vi "FPGA_EncoderReadConfiguration.vi"(8 "error in (no error)":errorcluster, 11 "EncoderDevRef":T5) -> (0 "error out":errorcluster, 1 "BSource":T1={"DevStatus"={"status"=FALSE, "code"=0, "source"=""}, "AnalogTriggerMode?"=FALSE, "DigitalMode"={"DIO Channel"=enum."Disabled"}, "AnalogTriggerMode"={"AnalogTriggerIndex"=enum."Trig 0", "OutputType"=enum."InWindow"}}, 2 "ASource":T1={"DevStatus"={"status"=FALSE, "code"=0, "source"=""}, "AnalogTriggerMode?"=FALSE, "DigitalMode"={"DIO Channel"=enum."Disabled"}, "AnalogTriggerMode"={"AnalogTriggerIndex"=enum."Trig 0", "OutputType"=enum."InWindow"}}, 3 "EncoderDevRef":T5, 4 "Reverse?":bool, 5 "IndexSource":T1={"DevStatus"={"status"=FALSE, "code"=0, "source"=""}, "AnalogTriggerMode?"=FALSE, "DigitalMode"={"DIO Channel"=enum."Disabled"}, "AnalogTriggerMode"={"AnalogTriggerIndex"=enum."Trig 0", "OutputType"=enum."InWindow"}}, 6 "IndexActiveHigh":bool, 7 "Enable":bool)   [LabVIEW 2017]
uses:
  <vilib>/Rock Robotics/SystemInterfaces/Encoder/FPGA_EncoderDevRef.ctl
  <vilib>/Rock Robotics/SystemInterfaces/Encoder/FPGA_EncoderIdx.ctl
  <vilib>/Rock Robotics/SystemInterfaces/CounterEncoderSourceConvertion/FPGA_CounterEncoderSourceConvertionLVSourceType.ctl
  <vilib>/Rock Robotics/SystemInterfaces/DIO/FPGA_DIODigitalSourceChannel.ctl
  <vilib>/Rock Robotics/SystemInterfaces/AnalogTrigger/FPGA_AnalogTriggerIndex.ctl
  <vilib>/Rock Robotics/SystemInterfaces/AnalogTrigger/FPGA_AnalogTriggerOutType.ctl
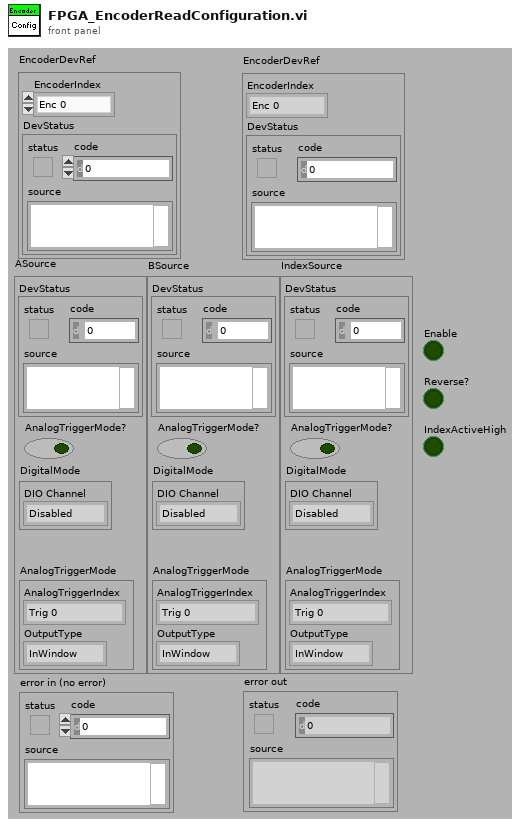
[diagram p1: front panel]
types:
  T1 = typedef "FPGA_CounterEncoderSourceConvertionLVSourceType.ctl" = cluster{"DevStatus":errorcluster, "AnalogTriggerMode?":bool, "DigitalMode":cluster{"DIO Channel":T2}, "AnalogTriggerMode":cluster{"AnalogTriggerIndex":T3, "OutputType":T4}}
  T2 = typedef "FPGA_DIODigitalSourceChannel.ctl" = enum8{"DIO 0", "DIO 1", "DIO 2", "DIO 3", "DIO 4", "DIO 5", "DIO 6", "DIO 7", "DIO 8", "DIO 9", "DIO MXP 0", "DIO MXP 1", "DIO MXP 2", "DIO MXP 3", "DIO MXP 4", "DIO MXP 5", "DIO MXP 6", "DIO MXP 7", "DIO MXP 8", "DIO MXP 9", "DIO MXP 10", "DIO MXP 11", "DIO MXP 12", "DIO MXP 13", "DIO MXP 14", "DIO MXP 15", "Disabled"}
  T3 = typedef "FPGA_AnalogTriggerIndex.ctl" = enum8{"Trig 0", "Trig 1", "Trig 2", "Trig 3", "Trig 4", "Trig 5", "Trig 6", "Trig 7", "Invalid"}
  T4 = typedef "FPGA_AnalogTriggerOutType.ctl" = enum16{"InWindow", "TriggerState", "Rising", "Falling"}
  T5 = typedef "FPGA_EncoderDevRef.ctl" = cluster{"EncoderIndex":T6, "DevStatus":errorcluster}
  T6 = typedef "FPGA_EncoderIdx.ctl" = enum8{"Enc 0", "Enc 1", "Enc 2", "Enc 3", "Enc 4", "Enc 5", "Enc 6", "Enc 7", "Invalid"}
  T7 = cluster{"ASource":cluster{"Channel":fxp<+,4,4>, "Module":fxp<+,1,1>, "AnalogTrigger":bool}, "BSource":cluster{"Channel":fxp<+,4,4>, "Module":fxp<+,1,1>, "AnalogTrigger":bool}, "IndexSource":cluster{"Channel":fxp<+,4,4>, "Module":fxp<+,1,1>, "AnalogTrigger":bool}, "IndexActiveHigh":bool, "Reverse":bool, "Enable":bool}
  T8 = cluster{"Channel":fxp<+,4,4>, "Module":fxp<+,1,1>, "AnalogTrigger":bool}
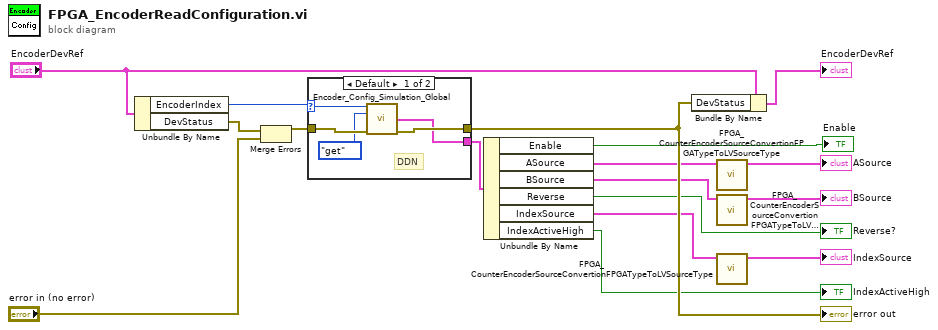
[diagram p0: block diagram]
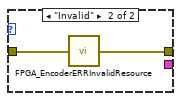
[diagram p2: hidden frame]
diagram:
  n1 = Unbundle By Name("EncoderDevRef") -> ("EncoderIndex"=w7:T6, "DevStatus"=w1:errorcluster)
  n2 = Merge Errors(w1, "error in (no error)") -> (w2:errorcluster)
  n3 = case shown="Default" w7 {
    selector: w7 -> [w22 _]
    tunnel: w2 -> [w21 w24]
    tunnel: [w20 w23] -> w14
    tunnel: [w19 _] -> w6
    frame Default {
      # "DDN"
      n4 = call <vilib>:"Encoder_Config_Simulation_Global.vi"("EncoderIndex"=w22, "menu"=enum16{"set", "get", "delete"}."get", "error in (no error)"=w21) -> ("Encoder Config get"=w19:T7, "error out"=w20:errorcluster)  [unwired: 11 in]
    }
    frame "Invalid" {
      n5 = call <vilib>:"FPGA_EncoderERRInvalidResource.vi"("error in (no error)"=w24) -> ("error out"=w23:errorcluster)
    }
  }
  "error out" <- w14
  n6 = Unbundle By Name(w6) -> ("Enable"=→"Enable":bool, "ASource"=w5:T8, "BSource"=w4:T8, "Reverse"=→"Reverse?":bool, "IndexSource"=w3:T8, "IndexActiveHigh"=→"IndexActiveHigh":bool)
  n7 = Bundle By Name(cluster="EncoderDevRef", "DevStatus"=w14) -> (→"EncoderDevRef":T5)
  n8 = call <vilib>:"FPGA_CounterEncoderSourceConvertionFPGATypeToLVSourceType.vi"("FPGASource"=w5) -> ("DigitalSource"=→"ASource":T1)  [unwired: 10 out]
  n9 = call <vilib>:"FPGA_CounterEncoderSourceConvertionFPGATypeToLVSourceType.vi"("FPGASource"=w4) -> ("DigitalSource"=→"BSource":T1)  [unwired: 10 out]
  n10 = call <vilib>:"FPGA_CounterEncoderSourceConvertionFPGATypeToLVSourceType.vi"("FPGASource"=w3) -> ("DigitalSource"=→"IndexSource":T1)  [unwired: 10 out]
